vi "Multiplication-Table.vi"() -> ()   [LabVIEW 2014]
panel:
  in  "number 2":i32
  in  "number 1":i32
  out "Table Control":string[][](table)
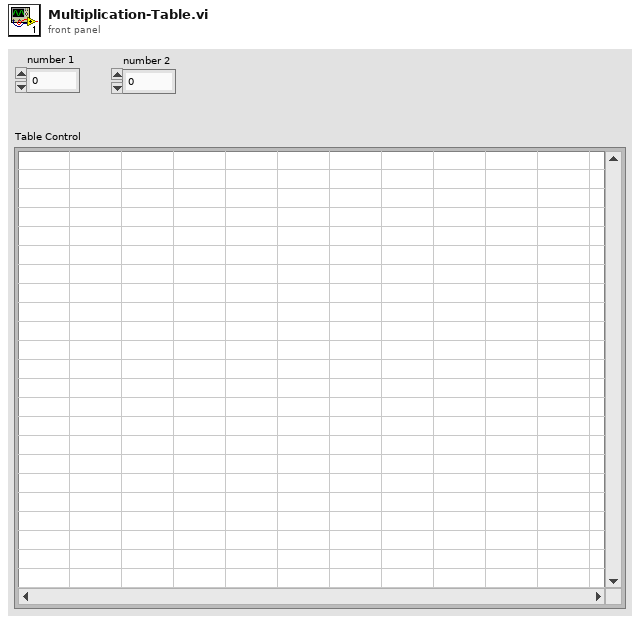
[diagram p1: front panel]
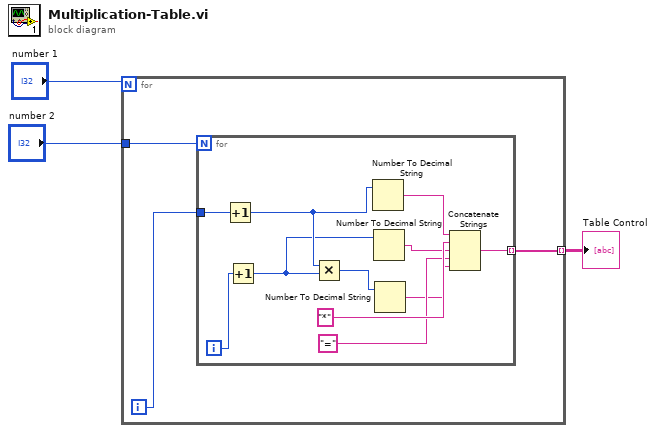
[diagram p0: block diagram]
diagram:
  n1 = for {
    N: "number 1" -> [_]
    tunnel: "number 2" -> [w6]
    tunnel: [w4] -> w1 mode=indexing
    i -> [w5]
    n2 = for {
      N: w6 -> [_]
      tunnel: w5 -> [w17]
      tunnel: [w10] -> w4 mode=indexing
      i -> [w16]
      n3 = Increment(x=w17) -> (x+1=w9:i32)
      n4 = Increment(x=w16) -> (x+1=w8:i32)
      n5 = Multiply(x=w9, y=w8) -> (x*y=w7:i32)
      n6 = Number To Decimal String(number=w9) -> (decimal integer string=w15:string)  [unwired: 1 in]
      n7 = Number To Decimal String(number=w8) -> (decimal integer string=w13:string)  [unwired: 1 in]
      n8 = Number To Decimal String(number=w7) -> (decimal integer string=w11:string)  [unwired: 1 in]
      n9 = Concatenate Strings(w15, "*", w13, "=", w11) -> (w10:string)
    }
  }
  "Table Control" <- w1
